vi "dfd_Render Transfer Function Equation.vi"(5 "fonts input":T3(array[cluster])=[{"Font Name:"="tahoma", "Size"=13, "Strikeout?"=FALSE, "Italic?"=FALSE, "Underline?"=FALSE, "Outline?"=TRUE, "Shadow?"=FALSE, "Bold?"=FALSE}, {"Font Name:"="tahoma", "Size"=13, "Strikeout?"=FALSE, "Italic?"=FALSE, "Underline?"=FALSE, "Outline?"=TRUE, "Shadow?"=FALSE, "Bold?"=FALSE}, {"Font Name:"="tahoma", "Size"=11, "Strikeout?"=FALSE, "Italic?"=FALSE, "Underline?"=FALSE, "Outline?"=TRUE, "Shadow?"=FALSE, "Bold?"=FALSE}], 6 "origin":cluster{"left":i16, "top":i16}, 7 "format coeffiecients":string="%#_g", 8 "error in":errorcluster, 9 "display format":u16(ring) items=["Expanded Form", " Second Order Sections"], 10 "filter coef":T1={"type"=enum."Undefined", "gain"=1.0, "coef a (k)"=[], "coef b (v)"=[]}, 11 "picture in":picture) -> (0 "error out":errorcluster, 1 "size":cluster{"width":i16, "height":i16}, 3 "picture out":picture)   [LabVIEW 2017, in "NI_DigFilter_Process.lvlib"]
uses:
  <vilib>/addons/Digital Filter Design/NI_DigFilter_Process.lvlib
  <vilib>/addons/Digital Filter Design/_Objects.llb/DFD Filter Coef.ctl
  <vilib>/addons/Digital Filter Design/_Objects.llb/DFD Filter Structure Type Selector.ctl
  <vilib>/addons/Digital Filter Design/NI_DigFilterLicensed.lvlib
panel:
  in  "variable":string="z"
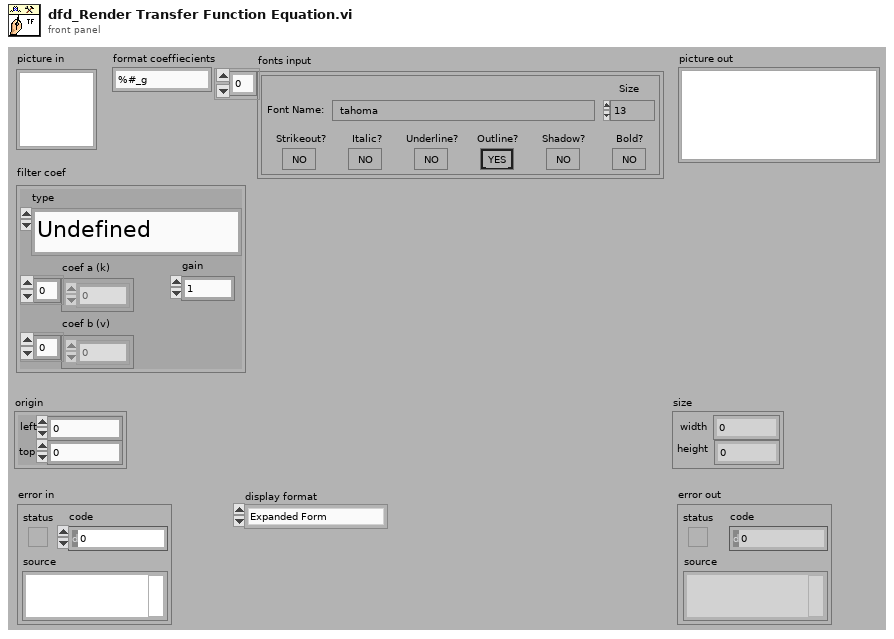
[diagram p1: front panel]
types:
  T1 = typedef "NI_DigFilterLicensed.lvlib/DFD Filter Coef.ctl" = cluster{"type":T2, "gain":dbl, "coef a (k)":dbl[], "coef b (v)":dbl[]}
  T2 = typedef "NI_DigFilterLicensed.lvlib/DFD Filter Structure Type Selector.ctl" = enum16{"Undefined", "FIR Direct Form", "FIR Direct Form Transposed", "FIR Symmetric", "FIR Antisymmetric", "IIR Direct Form I", "IIR Direct Form I Transposed", "IIR Direct Form II", "IIR Direct Form II Transposed", "IIR Cascaded Second Order Sections Form I", "IIR Cascaded Second Order Sections Form I Transposed", "IIR Cascaded Second Order Sections Form II", "IIR Cascaded Second Order Sections Form II Transposed", "Lattice Allpass (basic sections)", "Lattice Allpass (one multiplier sections)", "Lattice Allpass (normalized sections)", "Lattice AR (basic sections)", "Lattice AR (one multiplier sections)", "Lattice AR (normalized sections)", "Lattice MA (minimum phase)", "Lattice MA (maximum phase)", "Lattice ARMA (basic sections)", "Lattice ARMA (one multiplier sections)", "Lattice ARMA (normalized sections)"}
  T3 = cluster{"Font Name:":string, "Size":i16, "Strikeout?":bool, "Italic?":bool, "Underline?":bool, "Outline?":bool, "Shadow?":bool, "Bold?":bool}[]
  T4 = enum16{"User-specified Font", "Application Font", "System Font", "Dialog Font"}
  T5 = cluster{"coefficients ascending order":bool, "render ascending order":bool, "negative exponent":bool, "add bracket":bool}
  T6 = cluster{"horizontal":enum16{"left", "center", "right"}, "vertical":enum16{"top", "center", "bottom"}}
  T7 = cluster{"left":i16, "top":i16, "right":i16, "bottom":i16}
  T8 = cluster{"Font Name:":string, "Size":i16, "Strikeout?":bool, "Italic?":bool, "Underline?":bool, "Outline?":bool, "Shadow?":bool, "Bold?":bool}
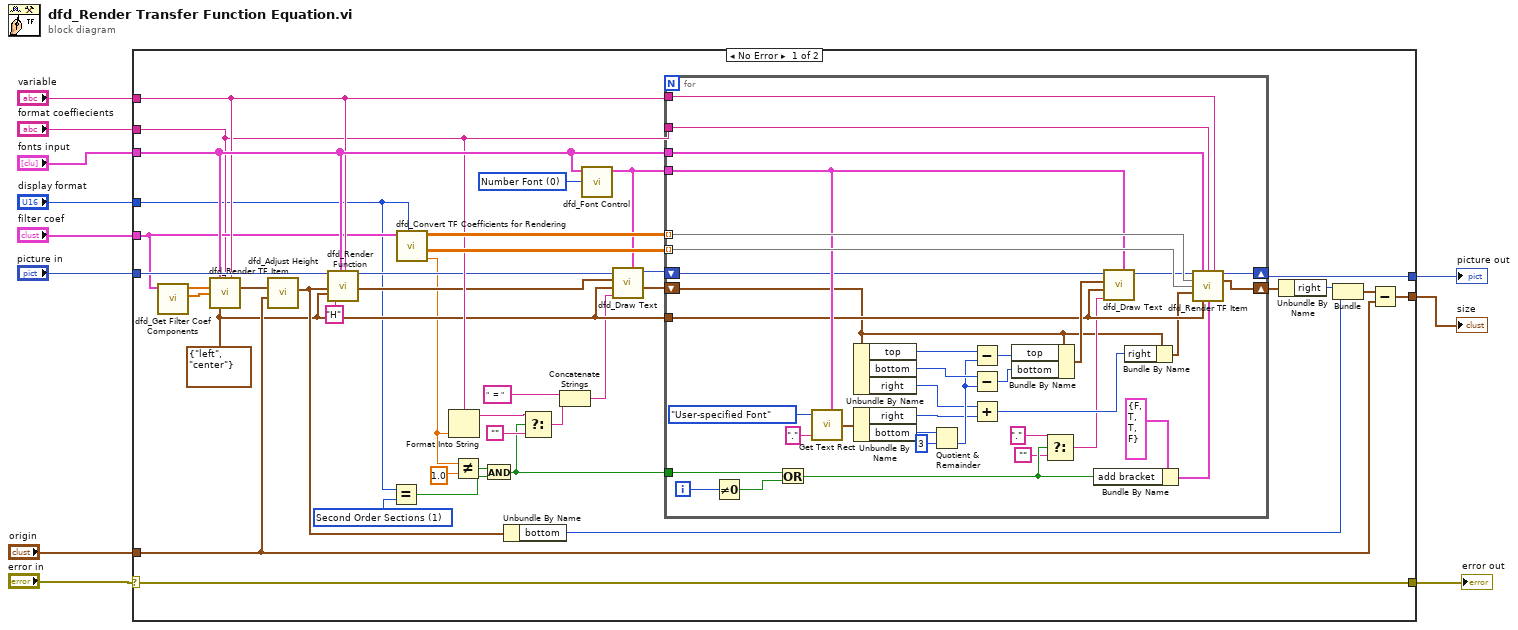
[diagram p0: block diagram]
diagram:
  n1 = case shown="No Error" "error in" {
    selector: "error in" -> [w47 w87]
    tunnel: "format coeffiecients" -> [w30 _]
    tunnel: "origin" -> [w36 _]
    tunnel: "picture in" -> [w49 _]
    tunnel: "variable" -> [w43 _]
    tunnel: "fonts input" -> [w44 _]
    tunnel: [w46 _] -> w1
    tunnel: "filter coef" -> [w33 _]
    tunnel: [w47 w87] -> w5
    tunnel: [w38 _] -> w4
    tunnel: "display format" -> [w23 _]
    frame No Error {
      w22 = u16 1 items=["Expanded Form", " Second Order Sections"] ("display format")
      w48 = u16 0 items=["Number Font", "Variable Font", "Script Font"] ("Tpye")
      w25 = T6 {"horizontal"=enum."left", "vertical"=enum."center"} ("alignment(left, top)")
      n2 = call <vilib>:"dfd_Get Filter Coef Components.vi"("filter coef"=w33) -> ("coef a (k)"=w31:dbl[], "coef b (v)"=w32:dbl[])  [unwired: 1 in, 8 out]
      n3 = call <vilib>:"dfd_Render TF Item.vi"("fonts input"=w44, "format coeffiecients"=w30, "variable"=w43, "numerator"=w32, "denominator"=w31, "alignment(left, top)"=w25) -> ("total rect"=w37:T7)  [unwired: 5 in, 4 out]
      n4 = call <vilib>:"dfd_Adjust Height.vi"("origin"=w36, "fraction rect"=w37) -> ("rect out"=w35:T7)  [unwired: 9 out]
      n5 = call <vilib>:"dfd_Render Function.vi"("picture"=w49, "rect in"=w35, "alignment(left, top)"=w25, "function name"="H", "fonts input"=w44, "variable"=w43) -> ("new picture"=w29:picture, "rect out"=w24:T7)  [unwired: 4 in, 8 out]
      n6 = Equal?(x=w23, y=w22) -> (x = y?=w18:bool)
      n7 = call <vilib>:"dfd_Convert TF Coefficients for Rendering.vi"("display format"=w23, "filter coef"=w33) -> ("gain"=w21:dbl, "denominator array"=w41:dbl[][], "numerator array"=w42:dbl[][])  [unwired: 2 in, 5 out]
      n8 = Format Into String(format string=w30, w21) -> (resulting string=w13:string)  [unwired: 2 in, 1 out]
      n9 = Not Equal?(x=w21, y=1.0) -> (x != y?=w19:bool)
      n10 = And(x=w19, y=w18) -> (x .and. y?=w14:bool)
      n11 = Unbundle By Name(w35) -> ("bottom"=w34:i16)
      n12 = Select(t=w13, s=w14, f="") -> (s? t:f=w15:string)
      n13 = Concatenate Strings("  = " ("text"), w15) -> (w12:string)
      n14 = call <vilib>:"dfd_Font Control.vi"("tpye"=w48, "fonts input"=w44) -> ("font output"=w27:T8)  [unwired: 9 out]
      n15 = call <vilib>:"dfd_Draw Text.vi"("font input"=w27, "text"=w12, "alignment(left, top)"=w25, "rect in"=w24, "picture in"=w29) -> ("rect out"=w26:T7, "picture out"=w28:picture)  [unwired: 3 in, 2 out]
      n16 = for {
        tunnel: w27 -> [w76]
        tunnel: w44 -> [w85]
        tunnel: w30 -> [w78]
        tunnel: w43 -> [w84]
        tunnel: w42 -> [w83] mode=indexing
        tunnel: w41 -> [w82] mode=indexing
        tunnel: w25 -> [w72]
        shift-right: [w86] -> w46
        shift-left: w28 -> [w55]
        shift-right: [w53] -> w45
        shift-left: w26 -> [w51]
        tunnel: w14 -> [w54]
        i -> [w81]
        n17 = Not Equal To 0?(x=w81) -> (x != 0?=w56:bool)
        n18 = Or(x=w54, y=w56) -> (x .or. y?=w60:bool)
        n19 = call <vilib>:"Get Text Rect.vi"("desired font(Application)"=T4."User-specified Font", "text"=".", "[user-specified font]"=w76) -> ("rect"=w71:T7)  [unwired: 3 in, 3 out]
        n20 = Unbundle By Name(w51) -> ("top"=w68:i16, "bottom"=w66:i16, "right"=w63:i16)
        n21 = Unbundle By Name(w71) -> ("right"=w62:i16, "bottom"=w70:i16)
        n22 = Quotient & Remainder(x=w70, y=i16 3) -> (floor(x/y)=w64:i16)  [unwired: 1 out]
        n23 = Subtract(x=w68, y=w64) -> (x-y=w67:i16)
        n24 = Subtract(x=w66, y=w64) -> (x-y=w65:i16)
        n25 = Add(x=w63, y=w62) -> (x+y=w61:i16)
        n26 = Bundle By Name(cluster=w51, "top"=w67, "bottom"=w65) -> (w73:T7)
        n27 = Select(t=".", s=w60, f="") -> (s? t:f=w59:string)
        n28 = Bundle By Name(cluster=T5 {"coefficients ascending order"=FALSE, "render ascending order"=TRUE, "negative exponent"=TRUE, "add bracket"=FALSE} ("rendering options"), "add bracket"=w60) -> (w79:T5)
        n29 = call <vilib>:"dfd_Draw Text.vi"("font input"=w76, "text"=w59, "alignment(left, top)"=w72, "rect in"=w73, "picture in"=w55) -> ("picture out"=w77:picture)  [unwired: 3 in, 3 out]
        n30 = Bundle By Name(cluster=w51, "right"=w61) -> (w52:T7)
        n31 = call <vilib>:"dfd_Render TF Item.vi"("picture in"=w77, "fonts input"=w85, "format coeffiecients"=w78, "variable"=w84, "numerator"=w83, "denominator"=w82, "rect in"=w52, "alignment(left, top)"=w72, "rendering options"=w79) -> ("picture out"=w86:picture, "total rect"=w53:T7)  [unwired: 2 in, 3 out]
      }
      n32 = Unbundle By Name(w45) -> ("right"=w40:i16)
      n33 = Bundle("right"=w40, "bottom"=w34) -> (w39:cluster{"right":i16, "bottom":i16})  [unwired: 1 out]
      n34 = Subtract(x=w39, y=w36) -> (x-y=w38:cluster{i16, i16})
    }
    frame Error {
    }
  }
  "picture out" <- w1
  "error out" <- w5
  "size" <- w4
